vi "From Variant.vi"(8 "error in (no error)":errorcluster, 11 "Variant":variant) -> (0 "error out":errorcluster, 3 "Boolean out":refnum<class "I32.lvclass">)   [LabVIEW 2017, in "I32.lvclass"]
uses:
  <vilib>/gpm_packages/@cs/data-type-serializer/source/I32/I32.lvclass
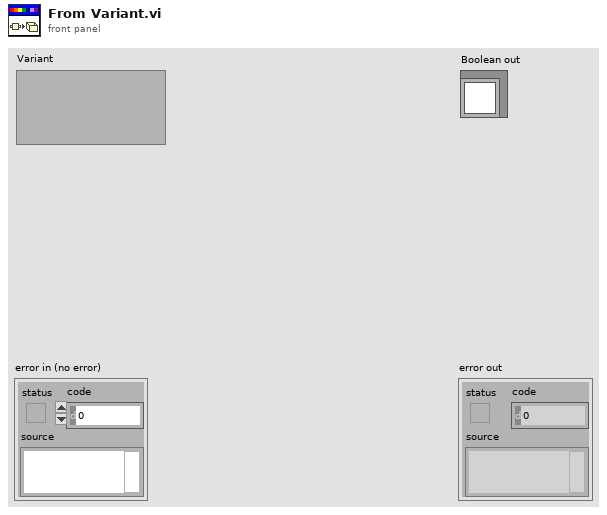
[diagram p1: front panel]
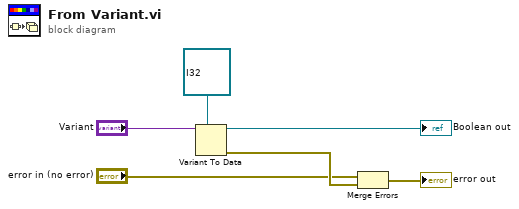
[diagram p0: block diagram]
diagram:
  n1 = Variant To Data(type=refnum<class "I32.lvclass"> refnum ("Boolean in"), Variant="Variant") -> (data=→"Boolean out":refnum<class "I32.lvclass">, error out=w5:errorcluster)  [unwired: 1 in]
  n2 = Merge Errors("error in (no error)", w5) -> (→"error out":errorcluster)
